vi "Get Gyro Sensor.vi"() -> (2 "Robot Field Orientation (deg)":dbl)   [LabVIEW 2018]
uses:
  <vilib>/Rock Robotics/Network Tables/NT Write Number.vi
  <vilib>/Rock Robotics/WPI/ThirdParty/Sensors/ADIS16448 IMU/ADIS16448_IMU.lvlib
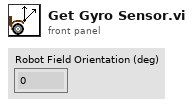
[diagram p1: front panel]
types:
  T1 = cluster{"Yaw":dbl, "Roll":dbl, "Pitch":dbl, "Heading":dbl, "Fused Heading":dbl}
  T2 = typedef "ADIS16448_IMU.lvlib/ADI_IMU_ADIS16448_IMUDevRef.ctl" = cluster{"DevStatus":errorcluster, "Handle":i32, "SPI Bus":T3, "Device Found":bool, "Device Ready":bool, "Yaw Axis":enum16{"X", "Y", "Z"}, "AHRS Algorithm":enum16{"Complementary", "Madgwick"}, "Serial":u16, "Lot ID 2":u16, "Lot ID 1":u16, "Bytes Per Sample":u16, "Calibrate On Open?":bool}
  T3 = typedef "spi_bus.ctl" = enum16{"SPI On-Board, CS0", "SPI On-Board, CS1", "SPI On-Board, CS2", "SPI On-Board, CS3", "SPI MXP", "Invalid"}
  T4 = cluster{"X Angle":dbl, "Y Angle":dbl, "Z Angle":dbl}
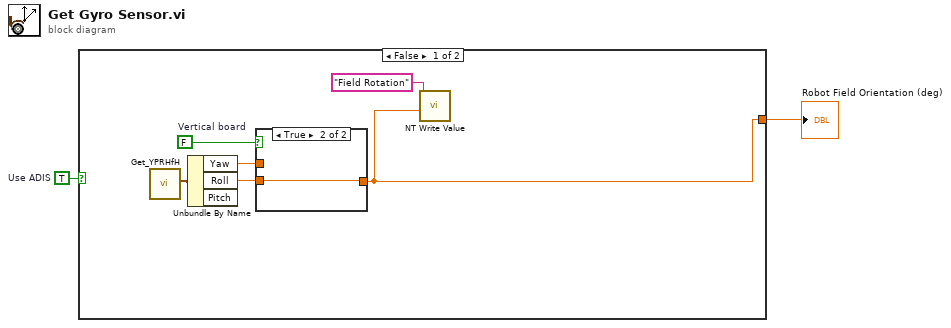
[diagram p0: block diagram]
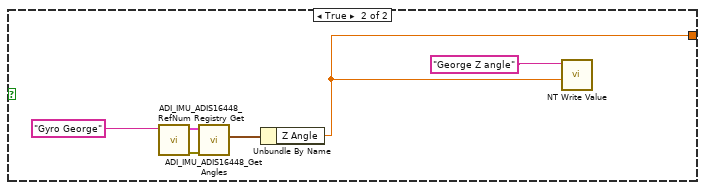
[diagram p3: hidden frame]
diagram:
  w1 = TRUE  # Use ADIS
  n1 = case shown="False" w1 {
    tunnel: [w3 w11] -> w2
    frame False {
      w6 = FALSE  # Vertical board
      n2 = call "Get_YPRHfH.vi"() -> ("YRPHfH"=w8:T1)  [unwired: 11 in]
      n3 = Unbundle By Name(w8) -> ("Yaw"=w5:dbl, "Roll"=w4:dbl)  [unwired: 1 out]
      n4 = case shown="True" w6 {
        tunnel: w5 -> [w9 _]
        tunnel: w4 -> [_ w10]
        tunnel: [w9 w10] -> w3
        frame False {
        }
        frame True {
        }
      }
      n5 = call-poly <vilib>:"NT Write Value.vi"("Numeric"=w3, "Name"="Field Rotation") -> ()  [unwired: 9 in, 1 out]
    }
    frame True {
      n6 = call <vilib>:"ADI_IMU_ADIS16448_RefNum Registry Get.vi"("refnum name"="Gyro George") -> ("error out"=w15:errorcluster, "ADI IMU DevRef"=w14:T2)  [unwired: 9 in]
      n7 = call <vilib>:"ADI_IMU_ADIS16448_Get Angles.vi"("error in"=w15, "ADI IMU DevRef"=w14) -> ("IMU Angles Out"=w12:T4)  [unwired: 6 in, 3 out]
      n8 = Unbundle By Name(w12) -> ("Z Angle"=w11:dbl)
      n9 = call-poly <vilib>:"NT Write Value.vi"("Numeric"=w11, "Name"="George Z angle") -> ()  [unwired: 9 in, 1 out]
    }
  }
  "Robot Field Orientation (deg)" <- w2
